vi "Force Extrema Set.vi"(8 "error in (no error)":errorcluster, 9 "Minimum Force":T1={"Fx (N)"=-3.0, "Fy (N)"=-3.0, "Fz (N)"=-3.0} {"Fx (N)" format="%.1f"; "Fy (N)" format="%.1f"; "Fz (N)" format="%.1f"}, 10 "Maximum Force":T1={"Fx (N)"=3.0, "Fy (N)"=3.0, "Fz (N)"=3.0} {"Fx (N)" format="%.1f"; "Fy (N)" format="%.1f"; "Fz (N)" format="%.1f"}) -> (0 "error out":errorcluster)   [LabVIEW 2019, in "Haptic Prog Interface.lvlib"]
doc: "Returns the forces of the haptic pen in N.\n\n<b>Position:</b> Returns a cluster of the x, y, and z forces on the pen (in units of N)."
uses:
  Haptic Prog Interface.lvlib
  dll_path.vi
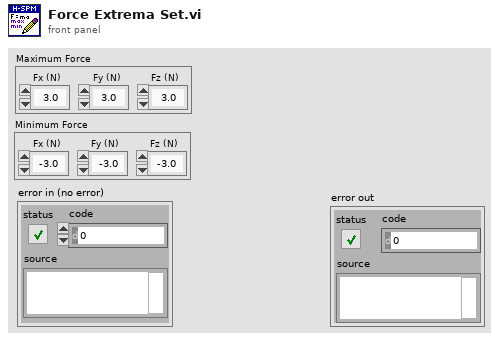
[diagram p1: front panel]
types:
  T1 = cluster{"Fx (N)":dbl, "Fy (N)":dbl, "Fz (N)":dbl}
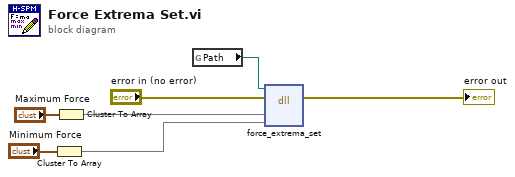
[diagram p0: block diagram]
diagram:
  n1 = Cluster To Array(cluster="Minimum Force") -> (array=w1:dbl[])
  n2 = Cluster To Array(cluster="Maximum Force") -> (array=w3:dbl[])
  n3 = global read "dll_path.vi" "Path"() -> (w7:path)
  n4 = dll-call lib="C:/Users/freem/Documents/GitHub/HapticSPM/Haptic-Programming-Interface/x64/Debug/Haptic Programming Interface.dll" fn="force_extrema_set"(path in=w7, error in="error in (no error)", "maxforce"=w3, "minforce"=w1) -> (error out=→"error out":errorcluster)  [unwired: 4 in, 1 out]
